vi "mapSensorIdToName.vi"(8 "error in (no error)":errorcluster, 10 "Sensor Id":i32[](array[numeric]), 11 "ZTAAC in":refnum<class "ZTAAC.lvclass">) -> (0 "error out":errorcluster, 1 "Sensor Num":i32, 2 "Sensor Name":string[](array[string]), 3 "ZTAAC out":refnum<class "ZTAAC.lvclass">)   [LabVIEW 2016, in "OfcFunc.lvlib" / "ZTAAC.lvclass"]
doc: "Map the array of sensor Id to sensor name."
uses:
  ZTAAC.lvclass
  ZTAAC.lvclass/ZTAAC.ctl
  MatOper/MatOper.lvclass
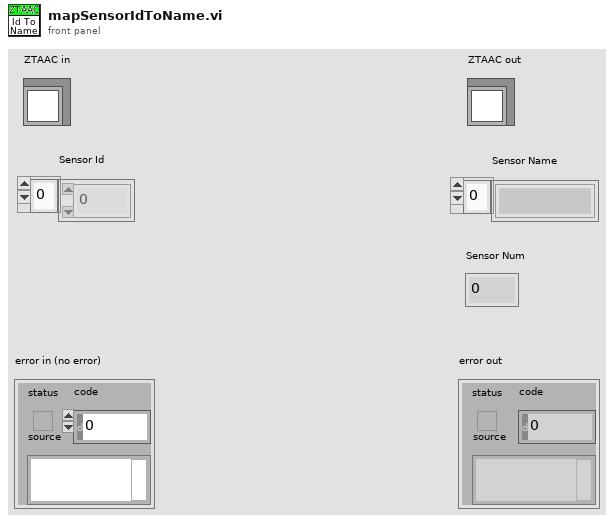
[diagram p1: front panel]
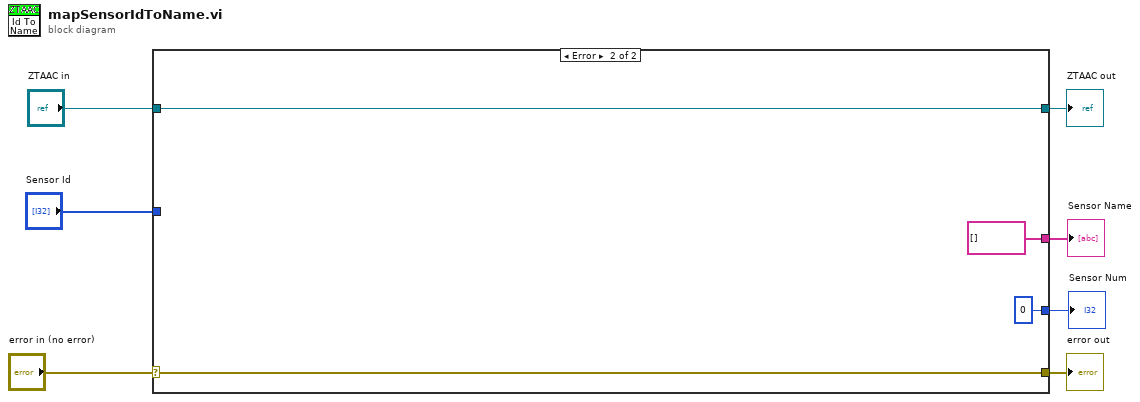
[diagram p0: block diagram]
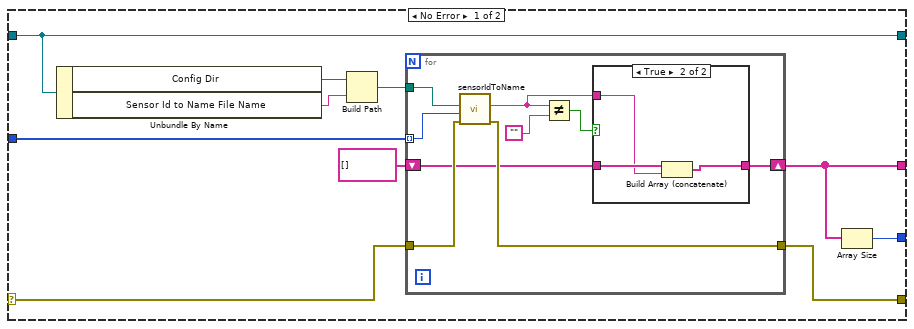
[diagram p2: hidden frame]
diagram:
  n1 = case shown="Error" "error in (no error)" {
    selector: "error in (no error)" -> [w12 w34]
    tunnel: [w11 w34] -> w6
    tunnel: [w17 w33] -> w4
    tunnel: "ZTAAC in" -> [w17 w33]
    tunnel: "Sensor Id" -> [w13 _]
    tunnel: [w9 string[] []] -> w2
    tunnel: [w8 0] -> w1
    frame No Error {
      n2 = Unbundle By Name(w17) -> ("Config Dir"=w16:path, "Sensor Id to Name File Name"=w15:string)
      n3 = Build Path(base path=w16, name or relative path=w15) -> (appended path=w14:path)
      n4 = for {
        tunnel: w14 -> [w26]
        tunnel: w13 -> [w25] mode=indexing
        tunnel: w12 -> [w24]
        tunnel: [w23] -> w11
        shift-right: [w19] -> w9
        shift-left: string[] [] -> [w20]
        n5 = call "sensorIdToName.vi"("error in (no error)"=w24, "Sensor ID"=w25, "Path"=w26) -> ("error out"=w23:errorcluster, "Sensor Name"=w18:string)  [unwired: 6 in, 1 out]
        n6 = Not Equal?(x=w18, y="") -> (x != y?=w21:bool)
        n7 = case shown="True" w21 {
          tunnel: w20 -> [w27 w30]
          tunnel: [w27 w29] -> w19
          tunnel: w18 -> [_ w28]
          frame False {
          }
          frame True {
            n8 = Build Array (concatenate)(w30, w28) -> (w29:string[])
          }
        }
      }
      n9 = Array Size(array=w9) -> (size(s)=w8:i32)
    }
    frame Error {
    }
  }
  "error out" <- w6
  "ZTAAC out" <- w4
  "Sensor Name" <- w2
  "Sensor Num" <- w1
